vi "ClimatronicsNamedSerial_get_rdg.vi"(4 "Channel Name":string, 7 "Address":T1={"Main"=61557, "Ch."=0, "Sub"=982, "Port Name"=""}) -> (0 "Output":dbl format="%.2f", 3 "Status note":string)   [LabVIEW 2018]
uses:
  ADAM Client/Sub VIs/ADAM Controls/Address.ctl
  ADAM Client/Sub VIs/ADAM Controls/Remember_value_mode.ctl
panel:
  out "Read":string="This is simulation mode"
  # "Channels:\n0: Velocity\n1: Direction\n2: Northerly\n3: Easterly\n4: Supply Volts\n5: 999Error\n6: ParseError\n7: SerialNo"
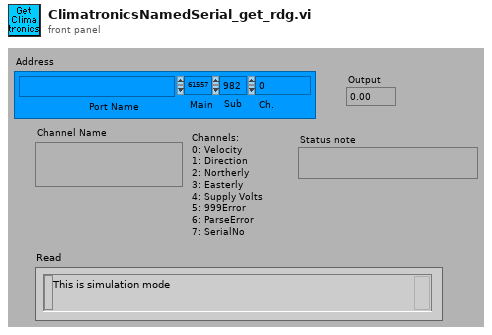
[diagram p1: front panel]
types:
  T1 = typedef "Address.ctl" = cluster{"Main":i32, "Ch.":i32, "Sub":i32, "Port Name":string}
  T2 = typedef "Remember_value_mode.ctl" = enum16{"Read only", "Read and Write"}
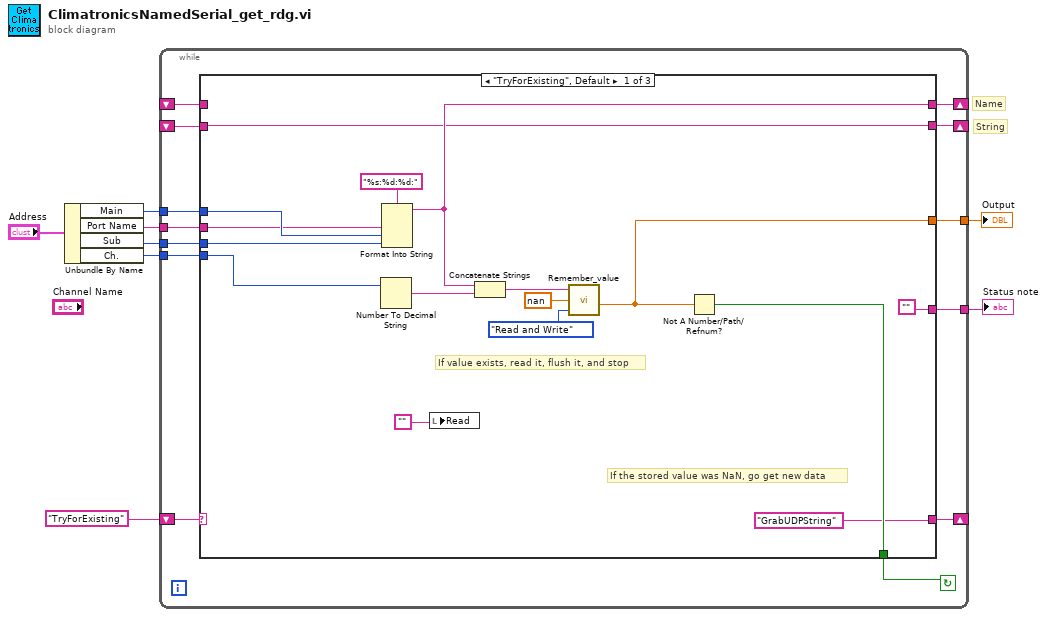
[diagram p0: block diagram]
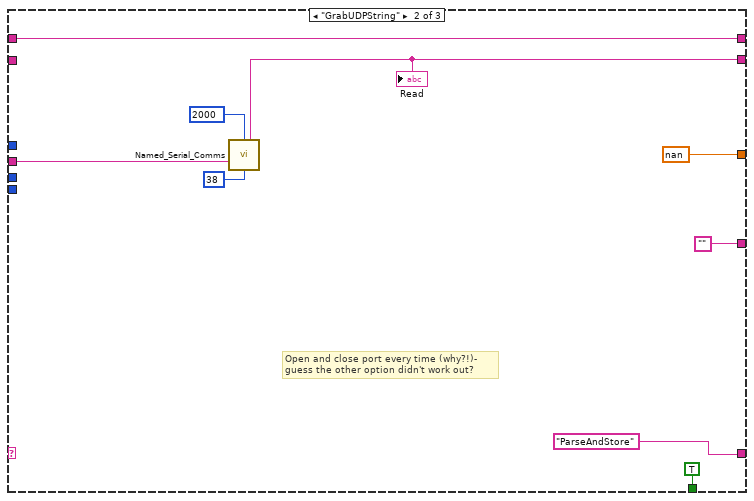
[diagram p2: hidden frame]
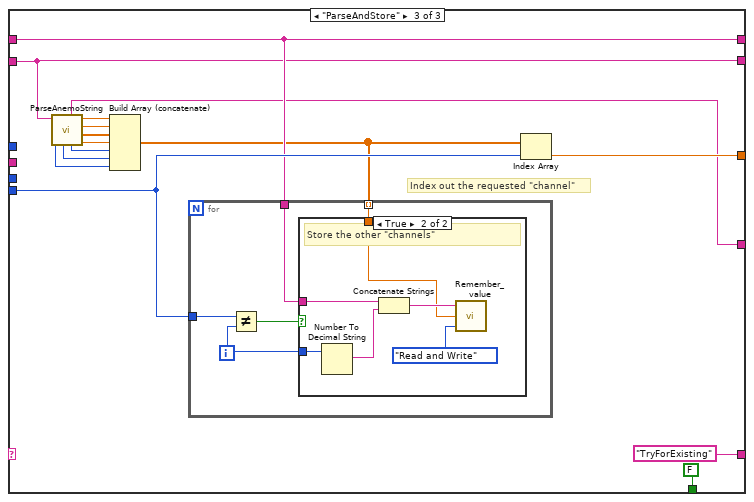
[diagram p3: hidden frame]
diagram:
  # "String"
  # "Name"
  n1 = Unbundle By Name("Address") -> ("Main"=w2:i32, "Port Name"=w7:string, "Sub"=w6:i32, "Ch."=w3:i32)
  n2 = while {
    shift-left: _ -> [w12]
    shift-right: [w13] -> _
    tunnel: [w15] -> w4
    tunnel: [w16] -> w5
    shift-left: _ -> [w11]
    shift-right: [w17] -> _
    shift-left: "TryForExisting" -> [w10]
    shift-right: [w9] -> _
    tunnel: w3 -> [w18]
    tunnel: w2 -> [w19]
    tunnel: w6 -> [w20]
    tunnel: w7 -> [w21]
    stop <- w14 continue-if-true
    n3 = case shown="\"TryForExisting\", Default" w10 {
      tunnel: w21 -> [w24 w42 _]
      tunnel: w20 -> [w36 _ _]
      tunnel: w19 -> [w37 _ _]
      tunnel: w18 -> [w34 _ w59]
      tunnel: ["GrabUDPString" "ParseAndStore" "TryForExisting"] -> w9
      tunnel: [w33 w45 w58] -> w17
      tunnel: [w26 nan w60] -> w16
      tunnel: ["" "" w47] -> w15
      tunnel: [w25 TRUE FALSE] -> w14
      tunnel: [w28 w41 w57] -> w13
      tunnel: w12 -> [w28 _ w57]
      tunnel: w11 -> [_ w45 w58]
      frame "TryForExisting", Default {
        # "If the stored value was NaN, go get new data"
        # "If value exists, read it, flush it, and stop"
        n4 = Number To Decimal String(number=w34) -> (decimal integer string=w32:string)  [unwired: 1 out]
        n5 = Format Into String(format string="%s:%d:%d:" ("Format String"), w24, w37, w36) -> (resulting string=w33:string)  [unwired: 2 in, 1 out]
        n6 = local write "Read"("") -> ()
        n7 = Concatenate Strings(w33, w32) -> (w31:string)
        n8 = call "Remember_value.vi"("Mode"=Remember_value_mode."Read and Write", "Input Value"=nan, "Ch name"=w31) -> ("Output Value"=w26:dbl)
        n9 = Not A Number/Path/Refnum?(number/path/refnum=w26) -> (NaN/Path/Refnum?=w25:bool)
      }
      frame "GrabUDPString" {
        # "Open and close port every time (why?!)-\nguess the other option didn't work out?"
        n10 = call "Named_Serial_Comms.vi"("Timeout/ms"=u32 2000, "Port Name"=w42, "Terminate Count"=38) -> ("Read"=w41:string)  [unwired: 9 in, 3 out]
        "Read" <- w41
      }
      frame "ParseAndStore" {
        # "Index out the requested \"channel\""
        n11 = call "ParseAnemoString.vi"("String"=w57) -> ("SupplyVolts"=w51:dbl, "N,E Components"=w52:dbl[], "direction"=w54:dbl, "speed"=w55:dbl, "999Error"=w50:i32, "Status"=w47:string, "ParseError"=w49:i32, "SerialNo"=w48:i32)  [unwired: 3 in]
        n12 = Build Array (concatenate)(w55, w54, w52, w51, w50, w49, w48) -> (w53:dbl[])
        n13 = for {
          tunnel: w58 -> [w66]
          tunnel: w53 -> [w65] mode=indexing
          tunnel: w59 -> [w63]
          i -> [w64]
          n14 = Not Equal?(x=w63, y=w64) -> (x != y?=w62:bool)
          n15 = case shown="True" w62 {
            tunnel: w64 -> [_ w72]
            tunnel: w66 -> [_ w70]
            tunnel: w65 -> [_ w67]
            frame False {
              # "Don't store the requested channel"
            }
            frame True {
              # "Store the other \"channels\""
              n16 = Number To Decimal String(number=w72) -> (decimal integer string=w71:string)  [unwired: 1 out]
              n17 = Concatenate Strings(w70, w71) -> (w68:string)
              n18 = call "Remember_value.vi"("Mode"=Remember_value_mode."Read and Write", "Input Value"=w67, "Ch name"=w68) -> ()  [unwired: 1 out]
            }
          }
        }
        n19 = Index Array(array=w53, index=w59) -> (element=w60:dbl)
      }
    }
  }
  "Output" <- w5
  "Status note" <- w4
